vi "Draw.vi"(2 "Number of decks":i32, 3 "Input used cards":i32[](array[numeric])) -> (0 "No. of card":i32, 1 "Output used cards":i32[](array[numeric]))   [LabVIEW 2018]
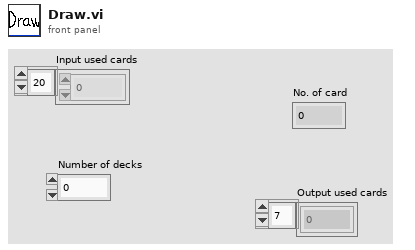
[diagram p1: front panel]
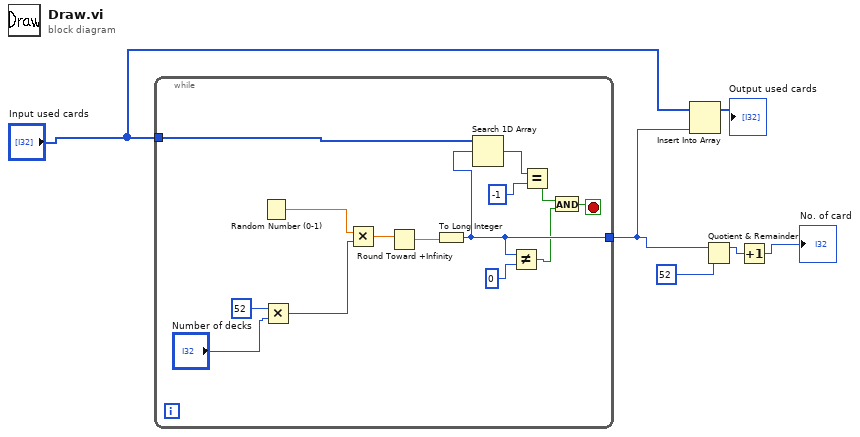
[diagram p0: block diagram]
diagram:
  n1 = while {
    tunnel: [w8] -> w5
    tunnel: "Input used cards" -> [w14]
    stop <- w11 stop-if-true
    n2 = Random Number (0-1)() -> (number: 0 to 1=w20:dbl)
    n3 = Multiply(x=52, y="Number of decks") -> (x*y=w17:i32)
    n4 = Multiply(x=w20, y=w17) -> (x*y=w16:dbl)
    n5 = Round Toward +Infinity(x=w16) -> (ceil(x): smallest int >= x=w15:dbl)
    n6 = To Long Integer(number=w15) -> (32bit integer=w8:i32)
    n7 = Search 1D Array(1D array=w14, element=w8) -> (index of element=w13:i32)  [unwired: 1 in]
    n8 = Not Equal?(x=w8, y=0) -> (x != y?=w7:bool)
    n9 = Equal?(x=w13, y=-1 ("元素索引")) -> (x = y?=w10:bool)
    n10 = And(x=w10, y=w7) -> (x .and. y?=w11:bool)
  }
  n11 = Insert Into Array(array="Input used cards", new element=w5) -> (→"Output used cards":i32[])  [unwired: 1 in]
  n12 = Quotient & Remainder(x=w5, y=52) -> (x-y*floor(x/y)=w2:i32)  [unwired: 1 out]
  n13 = Increment(x=w2) -> (x+1=→"No. of card":i32)
